vi "Parse Proto File.vi"(6 "Include Paths (None)":path[](array[path]), 8 "error in (no error)":errorcluster, 10 ".proto Path":path=path "C:/dev/proto/hello/hello.proto", 11 "ProtoParser in":refnum<class "ProtoParser.lvclass">) -> (0 "error out":errorcluster, 1 "Messages":map{string, T5}(c390), 2 "Enumerations":map{string, T1}(c390), 3 "ProtoParser out":refnum<class "ProtoParser.lvclass">)   [LabVIEW 2020, in "LV-Protoc.lvlib" / "ProtoParser.lvclass"]
uses:
  ProtoParser.lvclass
  LV-Proto/Message.ctl
  LV-Proto/Field.ctl
  LV-Proto/Type.ctl
  LV-Proto/Proto Type.ctl
  Raw Segment.ctl
  Segment Type.ctl
  LV-Proto/Enumeration.ctl
  LV-Proto/Enum Value.ctl
  Extract Segment.vi
  Strip Word.vi
  Consume Whitespace.vi
  Trim End.vi
  Strip To.vi
  Extract Enum Segments.vi
  LV-Proto/LV-Proto.lvlib
  LV-Protoc.lvlib
panel:
  out "Segments":T3[](array[typedef])
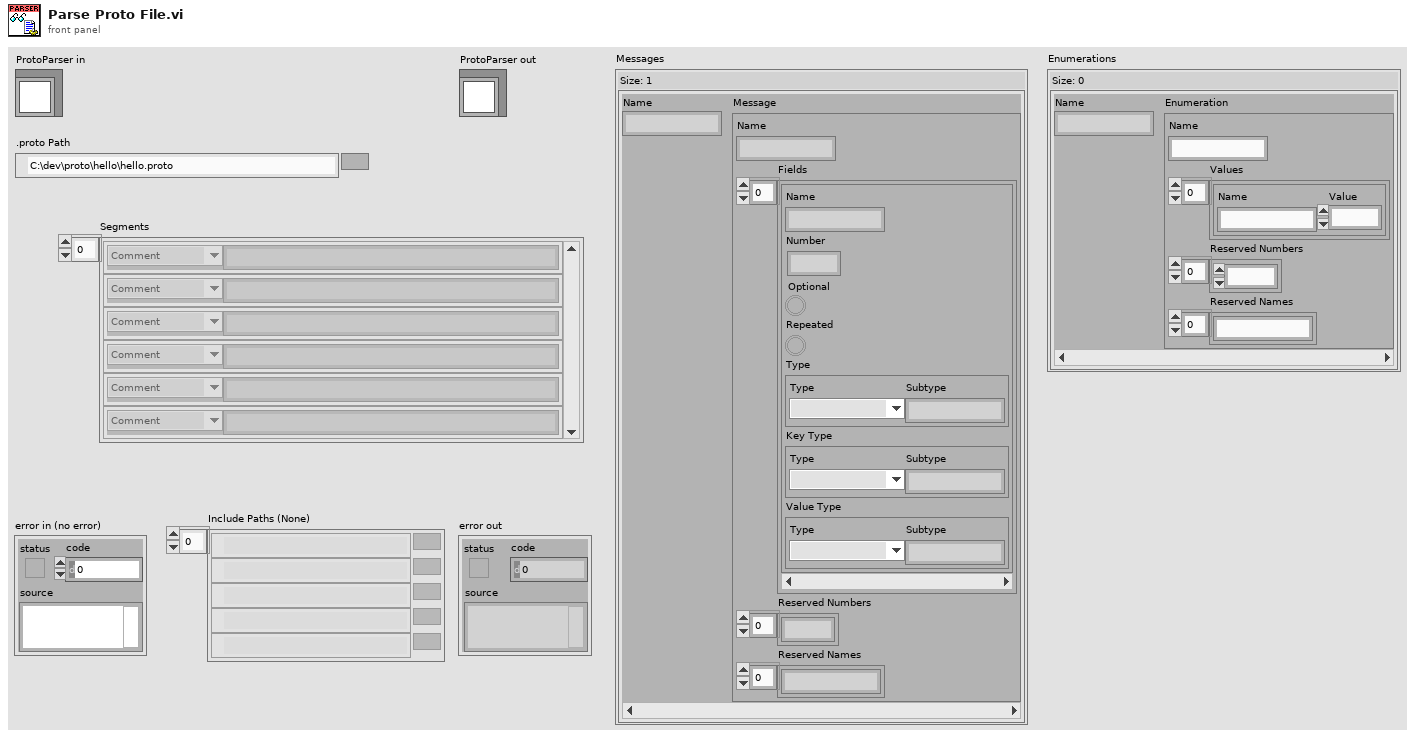
[diagram p1: front panel]
types:
  T1 = typedef "LV-Proto.lvlib/Enumeration.ctl" = cluster{"Name":string, "Values":T2[], "Reserved Numbers":u32[], "Reserved Names":string[]}
  T2 = typedef "LV-Proto.lvlib/Enum Value.ctl" = cluster{"Name":string, "Value":i32}
  T3 = typedef "LV-Protoc.lvlib/Raw Segment.ctl" = cluster{"Type":T4, "Text":string}
  T4 = typedef "LV-Protoc.lvlib/Segment Type.ctl" = enum16{"Comment", "Message Open", "Enum Open", "Message Close", "Enum Close", "Field", "Syntax", "Import", "Enum Value", "Package", "Reserved"}
  T5 = typedef "LV-Proto.lvlib/Message.ctl" = cluster{"Name":string, "Fields":T6[], "Reserved Numbers":u32[], "Reserved Names":string[]}
  T6 = typedef "LV-Proto.lvlib/Field.ctl" = cluster{"Name":string, "Number":u32, "Optional":bool, "Repeated":bool, "Type":T7, "Key Type":T7, "Value Type":T7}
  T7 = typedef "LV-Proto.lvlib/Type.ctl" = cluster{"Type":T8, "Subtype":string}
  T8 = typedef "LV-Proto.lvlib/Proto Type.ctl" = enum16{"UNKNOWN", "double", "float", "int32", "int64", "uint32", "uint64", "sint32", "sint64", "fixed32", "fixed64", "sfixed32", "sfixed64", "bool", "string", "bytes", "enum", "map", "message"}
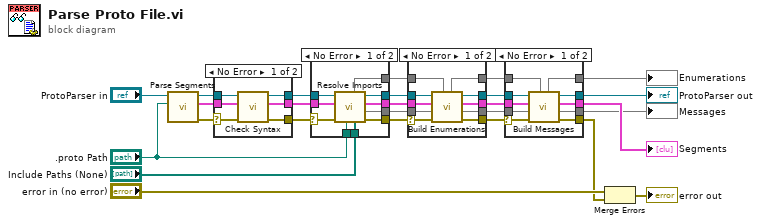
[diagram p0: block diagram]
diagram:
  n1 = call "Parse Segments.vi"("Proto Path"=".proto Path", "ProtoParser in"="ProtoParser in") -> ("error out"=w25:errorcluster, "Segments"=w21:T3[], "ProtoParser out"=w22:refnum<class "ProtoParser.lvclass">)  [unwired: 7 in]
  n2 = case shown="No Error" w25 {
    selector: w25 -> [w32 w33]
    tunnel: [w31 w33] -> w18
    tunnel: w22 -> [w30 w35]
    tunnel: [w29 w35] -> w20
    tunnel: w21 -> [w28 w34]
    tunnel: [w27 w34] -> w19
    frame No Error {
      n3 = call "Check Syntax.vi"("error in (no error)"=w32, "Segments in"=w28, "ProtoParser in"=w30) -> ("error out"=w31:errorcluster, "Segments"=w27:T3[], "ProtoParser out"=w29:refnum<class "ProtoParser.lvclass">)  [unwired: 5 in, 1 out]
    }
    frame Error {
    }
  }
  n4 = case shown="No Error" w18 {
    selector: w18 -> [w45 w46]
    tunnel: [w44 w46] -> w13
    tunnel: w20 -> [w43 w48]
    tunnel: [w42 w48] -> w15
    tunnel: w19 -> [w41 w47]
    tunnel: [w40 w47] -> w14
    tunnel: ".proto Path" -> [w39 _]
    tunnel: "Include Paths (None)" -> [w38 _]
    tunnel: [w37 _] -> w12
    tunnel: [w36 _] -> w11
    frame No Error {
      n5 = call "Resolve Imports.vi"("Include Paths"=w38, "Source .proto"=w39, "error in (no error)"=w45, "Segments in"=w41, "ProtoParser in"=w43) -> ("error out"=w44:errorcluster, "Messages"=w37:map{string, T5}, "Segments"=w40:T3[], "ProtoParser out"=w42:refnum<class "ProtoParser.lvclass">, "Enumerations"=w36:map{string, T1})  [unwired: 2 in]
    }
    frame Error {
    }
  }
  n6 = case shown="No Error" w13 {
    selector: w13 -> [w58 w59]
    tunnel: [w57 w59] -> w6
    tunnel: w15 -> [w56 w61]
    tunnel: [w55 w61] -> w9
    tunnel: w14 -> [w54 w60]
    tunnel: [w53 w60] -> w8
    tunnel: [w52 _] -> w7
    tunnel: [w51 _] -> w10
    tunnel: w12 -> [w50 _]
    tunnel: w11 -> [w49 _]
    frame No Error {
      n7 = call "Build Enumerations.vi"("Enumerations in"=w49, "error in (no error)"=w58, "Messages in"=w50, "Segments in"=w54, "ProtoParser in"=w56) -> ("error out"=w57:errorcluster, "Messages"=w52:map{string, T5}, "Segments"=w53:T3[], "ProtoParser out"=w55:refnum<class "ProtoParser.lvclass">, "Enumerations"=w51:map{string, T1})  [unwired: 2 in]
    }
    frame Error {
    }
  }
  n8 = case shown="No Error" w6 {
    selector: w6 -> [w71 w72]
    tunnel: [w70 w72] -> w1
    tunnel: w9 -> [w69 w74]
    tunnel: [w68 w74] -> w5
    tunnel: w8 -> [w67 w73]
    tunnel: [w66 w73] -> w26
    tunnel: [w65 _] -> w4
    tunnel: [w64 _] -> w3
    tunnel: w7 -> [w63 _]
    tunnel: w10 -> [w62 _]
    frame No Error {
      n9 = call "Build Messages.vi"("Enumerations in"=w62, "error in (no error)"=w71, "Messages in"=w63, "Segments in"=w67, "ProtoParser in"=w69) -> ("error out"=w70:errorcluster, "Messages"=w65:map{string, T5}, "Segments"=w66:T3[], "ProtoParser out"=w68:refnum<class "ProtoParser.lvclass">, "Enumerations"=w64:map{string, T1})  [unwired: 2 in]
    }
    frame Error {
    }
  }
  "ProtoParser out" <- w5
  "Messages" <- w4
  "Segments" <- w26
  "Enumerations" <- w3
  n10 = Merge Errors("error in (no error)", w1) -> (→"error out":errorcluster)
